vi "STT_STP_STEP_LMT_CHK.vi"(1 "Start":dbl=10000000.0, 2 "Stop":dbl=10000000.0, 3 "Step":dbl=10000000.0, 5 "error in":errorcluster) -> (14 "error out":errorcluster, 15 "Start":dbl=10000000.0, 16 "Stop":dbl=10000000.0, 17 "Step":dbl=10000000.0)   [LabVIEW 2018, in "PNA-X.lvlib"]
uses:
  PNA-X.lvlib
panel:
  out "Npoints":dbl=480.0
  in  "Npoints":dbl=1.0
  in  "Limits":T1={"SttMax"=26500000000.0, "SttMin"=10000000.0, "StpMax"=26500000000.0, "StpMin"=10000000.0, "StepMax"=26500000000.0, "StepMin"=10000000.0, "NpntsMax"=16001.0, "NpntsMin"=1.0}
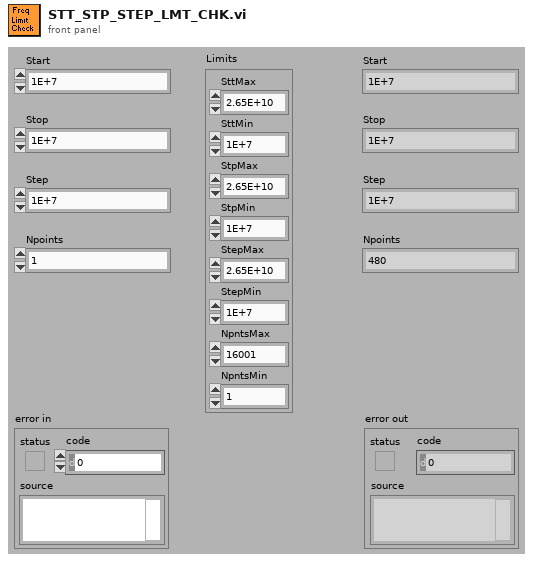
[diagram p1: front panel]
types:
  T1 = cluster{"SttMax":dbl, "SttMin":dbl, "StpMax":dbl, "StpMin":dbl, "StepMax":dbl, "StepMin":dbl, "NpntsMax":dbl, "NpntsMin":dbl}
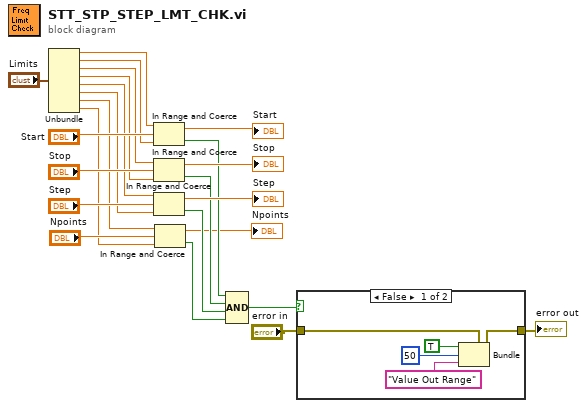
[diagram p0: block diagram]
diagram:
  n1 = Unbundle("Limits") -> ("SttMax"=w10:dbl, "SttMin"=w11:dbl, "StpMax"=w12:dbl, "StpMin"=w13:dbl, "StepMax"=w14:dbl, "StepMin"=w15:dbl, "NpntsMax"=w2:dbl, "NpntsMin"=w1:dbl)
  n2 = In Range and Coerce(upper limit=w10, x="Start", lower limit=w11) -> (coerced(x)=→"Start":dbl, In Range?=w9:bool)
  n3 = In Range and Coerce(upper limit=w12, x="Stop", lower limit=w13) -> (coerced(x)=→"Stop":dbl, In Range?=w8:bool)
  n4 = In Range and Coerce(upper limit=w14, x="Step", lower limit=w15) -> (coerced(x)=→"Step":dbl, In Range?=w7:bool)
  n5 = In Range and Coerce(upper limit=w2, x="Npoints", lower limit=w1) -> (coerced(x)=→"Npoints":dbl, In Range?=w3:bool)
  n6 = Compound Arithmetic op=AND(w9, w8, w7, w3) -> (w6:bool)
  n7 = case shown="False" w6 {
    tunnel: "error in" -> [w28 w30]
    tunnel: [w29 w30] -> w23
    frame False {
      n8 = Bundle(cluster=w28, "status"=TRUE, "code"=50, "source"="Value Out Range") -> (w29:errorcluster)
    }
    frame True {
    }
  }
  "error out" <- w23
